vi "ArrayBandpass.vi"(3 "Frequency":u32, 5 "Input":fxp<+/-,16,4>[](array[numeric])) -> (1 "Output":fxp<+/-,16,4>[](array[numeric]))   [LabVIEW 2015]
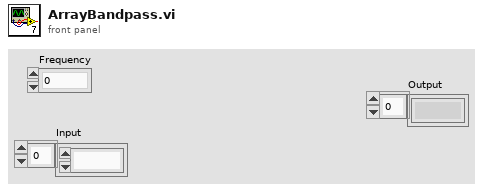
[diagram p1: front panel]
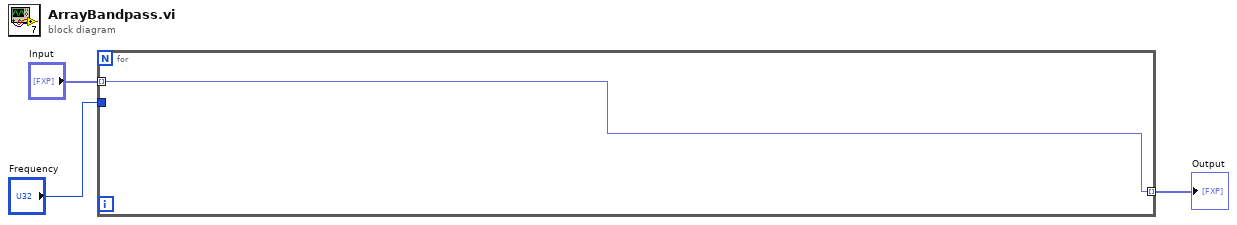
[diagram p0: block diagram]
diagram:
  n1 = for {
    tunnel: "Input" -> [w4] mode=indexing
    tunnel: "Frequency" -> [_]
    tunnel: [w4] -> w1 mode=indexing
  }
  "Output" <- w1
